vi "setParametresEssai.vi"(8 "error in (no error)":errorcluster, 10 "param":T1, 11 "VISA resource name":refnum<visa-resource-name>) -> (0 "error out":errorcluster, 3 "VISA resource name out":refnum<visa-resource-name>)   [LabVIEW 2023]
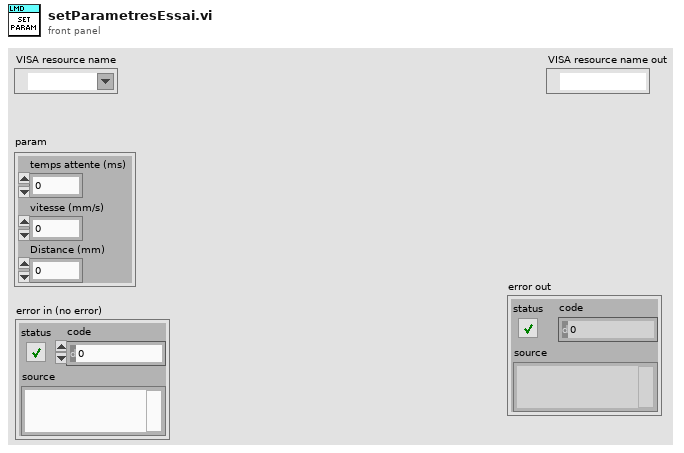
[diagram p1: front panel]
types:
  T1 = cluster{"temps attente (ms)":i32, "vitesse (mm/s)":dbl, "Distance (mm)":dbl}
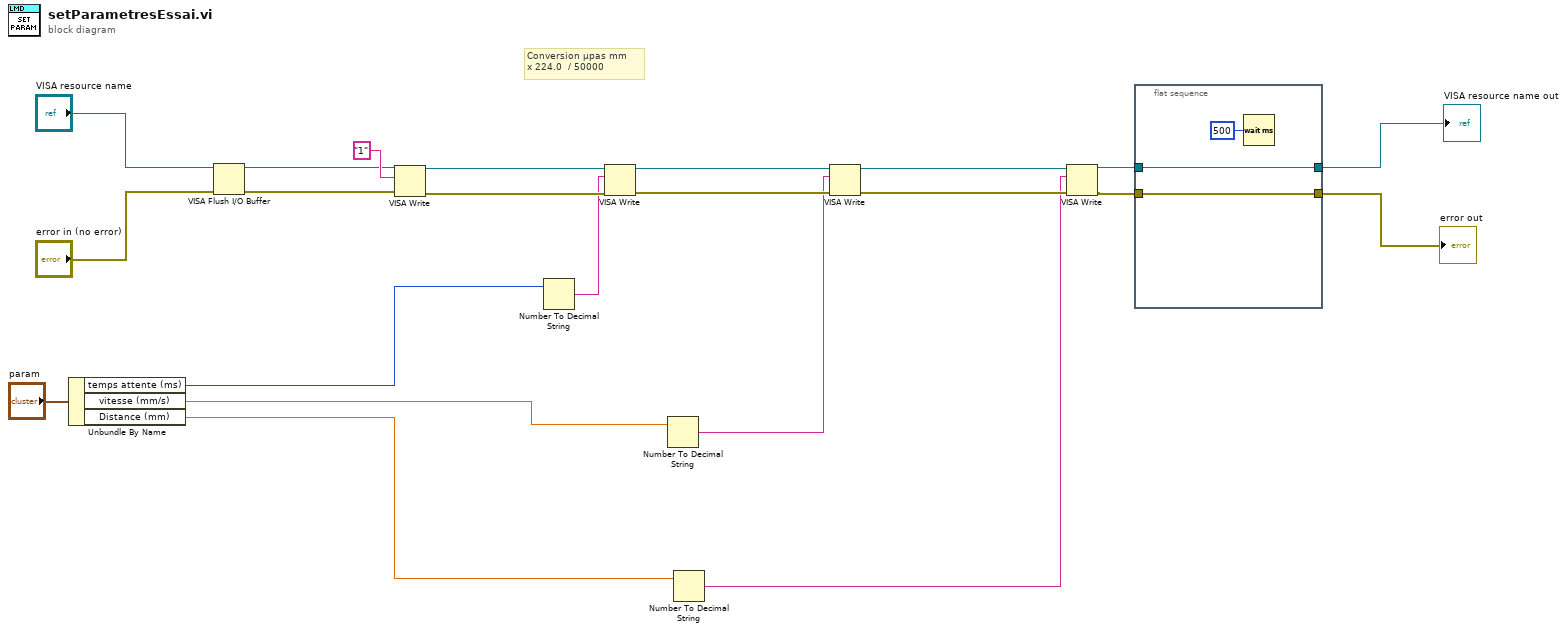
[diagram p0: block diagram]
diagram:
  # "Conversion µpas mm \nx 224.0  / 50000"
  n1 = Unbundle By Name("param") -> ("temps attente (ms)"=w20:i32, "vitesse (mm/s)"=w2:dbl, "Distance (mm)"=w1:dbl)
  n2 = VISA Flush I/O Buffer(VISA resource name="VISA resource name", error in (no error)="error in (no error)") -> (VISA resource name out=w10:refnum<visa-resource-name>, error out=w11:errorcluster)  [unwired: 1 in]
  n3 = VISA Write(VISA resource name=w10, write buffer="1", error in (no error)=w11) -> (VISA resource name out=w19:refnum<visa-resource-name>, error out=w18:errorcluster)  [unwired: 1 out]
  n4 = Number To Decimal String(number=w20) -> (decimal integer string=w9:string)  [unwired: 1 in]
  n5 = VISA Write(VISA resource name=w19, write buffer=w9, error in (no error)=w18) -> (VISA resource name out=w16:refnum<visa-resource-name>, error out=w17:errorcluster)  [unwired: 1 out]
  n6 = Number To Decimal String(number=w2) -> (decimal integer string=w8:string)  [unwired: 1 in]
  n7 = Number To Decimal String(number=w1) -> (decimal integer string=w7:string)  [unwired: 1 in]
  n8 = VISA Write(VISA resource name=w16, write buffer=w8, error in (no error)=w17) -> (VISA resource name out=w15:refnum<visa-resource-name>, error out=w14:errorcluster)  [unwired: 1 out]
  n9 = VISA Write(VISA resource name=w15, write buffer=w7, error in (no error)=w14) -> (VISA resource name out=w4:refnum<visa-resource-name>, error out=w5:errorcluster)  [unwired: 1 out]
  n10 = flat-sequence {
    tunnel: [w25] -> w6
    tunnel: w5 -> [w25]
    tunnel: w4 -> [w24]
    tunnel: [w24] -> w3
    frame #0 {
      n11 = Wait (ms)(milliseconds to wait=u32 500) -> ()  [unwired: 1 out]
    }
  }
  "error out" <- w6
  "VISA resource name out" <- w3
